vi "Selftest Device.vi"(8 "error in (no error)":errorcluster, 11 "IVI_Counter in":refnum<class "IVI_Counter.lvclass">) -> (0 "error out":errorcluster, 1 "Self-Test Result Message":string, 2 "Self-Test Result Code":i32, 3 "IVI_Counter out":refnum<class "IVI_Counter.lvclass">)   [LabVIEW 2013, in "IVI_Counter.lvlib" / "IVI_Counter.lvclass"]
doc: "Perform selftest of device."
uses:
  IVI_Counter.lvclass
  IVI_Counter.lvclass/IVI_Counter.ctl
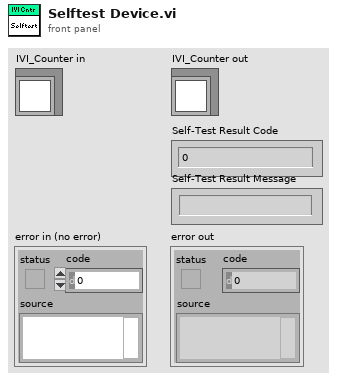
[diagram p1: front panel]
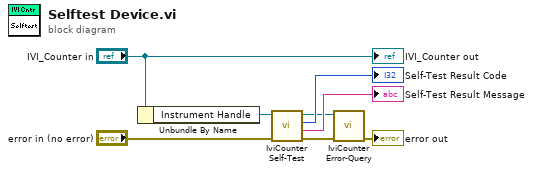
[diagram p0: block diagram]
diagram:
  n1 = Unbundle By Name("IVI_Counter in") -> ("Instrument Handle"=w7:refnum<k15>)
  n2 = call <vilib>:"IviCounter Self-Test.vi"("error in (no error)"="error in (no error)", "instrument handle"=w7) -> ("error out"=w3:errorcluster, "self-test message"=→"Self-Test Result Message":string, "self test result"=→"Self-Test Result Code":i16, "instrument handle out"=w1:refnum<k15>)  [unwired: 6 in]
  n3 = call <vilib>:"IviCounter Error-Query.vi"("error in (no error)"=w3, "instrument handle"=w1) -> ("error out"=→"error out":errorcluster)  [unwired: 6 in, 3 out]
  "IVI_Counter out" <- "IVI_Counter in"
